vi "Construct Storage Line Set (Implies).vi"() -> ()   [LabVIEW 2015]
panel:
  out "Include":bool
  in  "Clean":bool
  in  "Empty":bool
  in  "Numeric":u16
  out "number":u16
  in  "Boolean array":bool[](array[boolean])
  out ".not. x?":bool[](array[boolean])
  out "Open some":bool
  out "Close some":bool
  out "x .and. y?":bool[](array[boolean])
  in  "Control":bool[](array[boolean])
  in  "State":bool[](array[boolean])
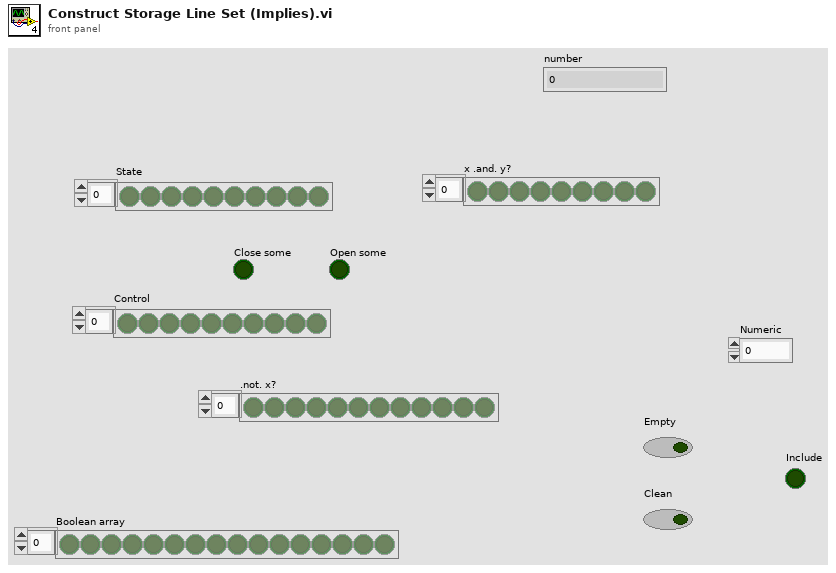
[diagram p1: front panel]
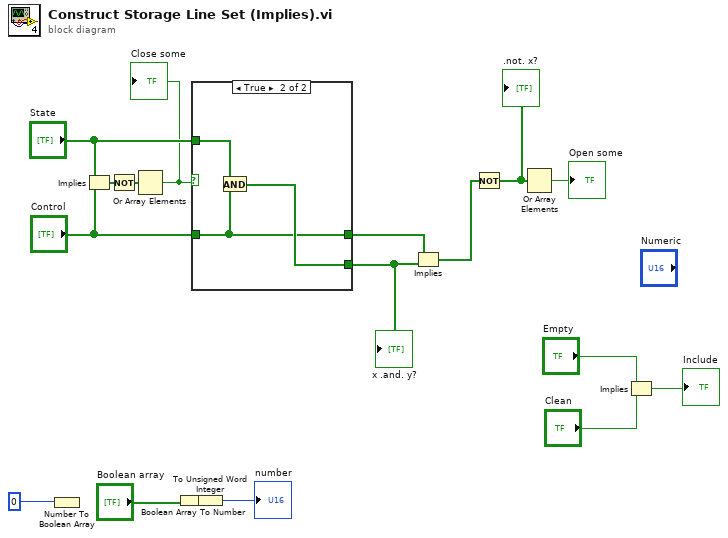
[diagram p0: block diagram]
diagram:
  n1 = Number To Boolean Array(number=u16 0) -> ()  [unwired: 1 out]
  n2 = Implies(1:"Control", 2:"State") -> (0:w16:bool[])
  n3 = Not(x=w16) -> (.not. x?=w15:bool[])
  n4 = Or Array Elements(Boolean array=w15) -> (logical OR=w9:bool)
  "Close some" <- w9
  n5 = Boolean Array To Number(Boolean array="Boolean array") -> (number=w5:u32)
  n6 = case shown="True" w9 {
    tunnel: [w18 w22] -> w17
    tunnel: "Control" -> [w19 w20]
    tunnel: "State" -> [w18 w21]
    tunnel: [w19 w20] -> w8
    frame False {
    }
    frame True {
      n7 = And(x=w21, y=w20) -> (x .and. y?=w22:bool[])
    }
  }
  "x .and. y?" <- w17
  n8 = To Unsigned Word Integer(number=w5) -> (unsigned 16bit integer=→"number":u16)
  n9 = Implies(1:w17, 2:w8) -> (0:w11:bool[])
  n10 = Not(x=w11) -> (.not. x?=w12:bool[])
  ".not. x?" <- w12
  n11 = Or Array Elements(Boolean array=w12) -> (logical OR=→"Open some":bool)
  n12 = Implies(1:"Clean", 2:"Empty") -> (0:→"Include":bool)
